vi "M--front LSw.vi"(8 "Command Info In":T2, 10 "M--front LSw":T1) -> (0 "Command Info Out":T2)   [LabVIEW 2017]
uses:
  <vilib>/Rock Robotics/WPI/Framework/Command Status Info.ctl
  <vilib>/Rock Robotics/WPI/Framework/Completion Status.ctl
  <vilib>/Rock Robotics/WPI/Framework/Completion Notifier.ctl
  Block Clusters/M--front LSw.ctl
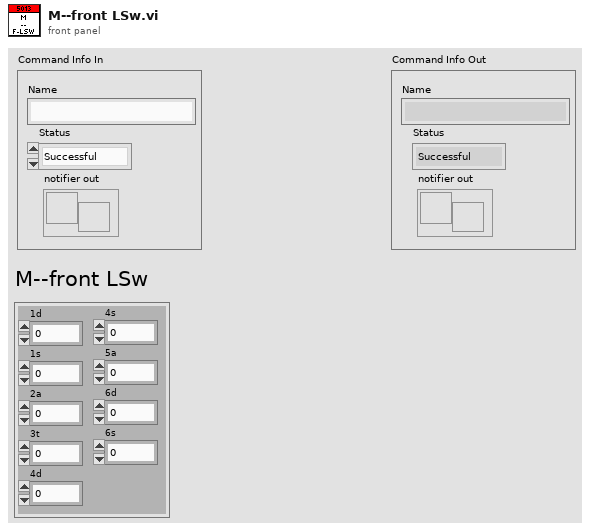
[diagram p1: front panel]
types:
  T1 = typedef "M--front LSw.ctl" = cluster{"1d":dbl, "1s":dbl, "2a":dbl, "3t":dbl, "4d":dbl, "4s":dbl, "5a":dbl, "6d":dbl, "6s":dbl}
  T2 = typedef "Command Status Info.ctl" = cluster{"Name":string, "Status":T3, "notifier out":T4}
  T3 = typedef "Completion Status.ctl" = enum16{"Successful", "Aborted", "Incomplete"}
  T4 = typedef "Completion Notifier.ctl" = refnum<notifier>
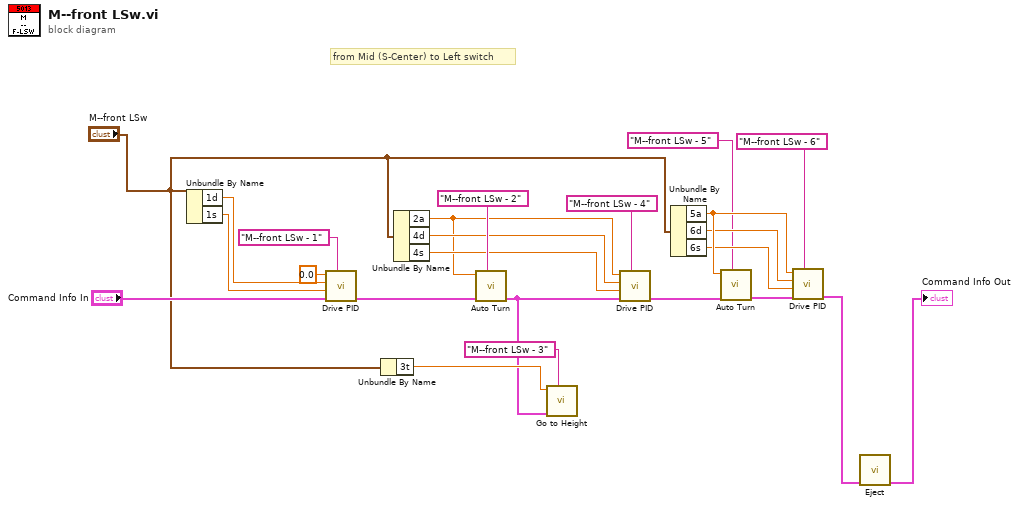
[diagram p0: block diagram]
diagram:
  # "from Mid (S-Center) to Left switch"
  n1 = Unbundle By Name("M--front LSw") -> ("1d"=w24:dbl, "1s"=w23:dbl)
  n2 = call "Drive PID.vi"("Description"="M--front LSw - 1", "Command Info In"="Command Info In", "Speed"=w23, "Distance"=w24, "Target Angle"=0.0) -> ("Command Info Out"=w18:T2)  [unwired: 6 in]
  n3 = Unbundle By Name("M--front LSw") -> ("3t"=w16:dbl)
  n4 = Unbundle By Name("M--front LSw") -> ("2a"=w9:dbl, "4d"=w13:dbl, "4s"=w12:dbl)
  n5 = call "Auto Turn.vi"("Description"="M--front LSw - 2", "Command Info In"=w18, "Target Angle"=w9) -> ("Command Info Out"=w14:T2)  [unwired: 8 in]
  n6 = call "Go to Height.vi"("Description"="M--front LSw - 3", "Command Info In"=w14, "Target Height (in)"=w16) -> ()  [unwired: 8 in, 1 out]
  n7 = call "Drive PID.vi"("Description"="M--front LSw - 4", "Command Info In"=w14, "Speed"=w12, "Distance"=w13, "Target Angle"=w9) -> ("Command Info Out"=w10:T2)  [unwired: 6 in]
  n8 = Unbundle By Name("M--front LSw") -> ("5a"=w6:dbl, "6d"=w5:dbl, "6s"=w4:dbl)
  n9 = call "Auto Turn.vi"("Description"="M--front LSw - 5", "Command Info In"=w10, "Target Angle"=w6) -> ("Command Info Out"=w7:T2)  [unwired: 8 in]
  n10 = call "Drive PID.vi"("Description"="M--front LSw - 6", "Command Info In"=w7, "Speed"=w4, "Distance"=w5, "Target Angle"=w6) -> ("Command Info Out"=w1:T2)  [unwired: 6 in]
  n11 = call "Eject.vi"("Command Info In"=w1) -> ("Command Info Out"=→"Command Info Out":T2)  [unwired: 10 in]
